vi "leapdata to fingers.vi"(11 "leapdata in":string="TYPE_THUMB0\nTYPE_INDEX72\nTYPE_MIDDLE67\nTYPE_RING57\nTYPE_PINKY59\n" caption="字符串/二进制数据") -> (1 "Recognize  hands":T1, 3 "fingerdata":T2)   [LabVIEW 2016]
uses:
  Controls/recognize hands data.ctl
panel:
  out "数字":i32[](array[numeric])
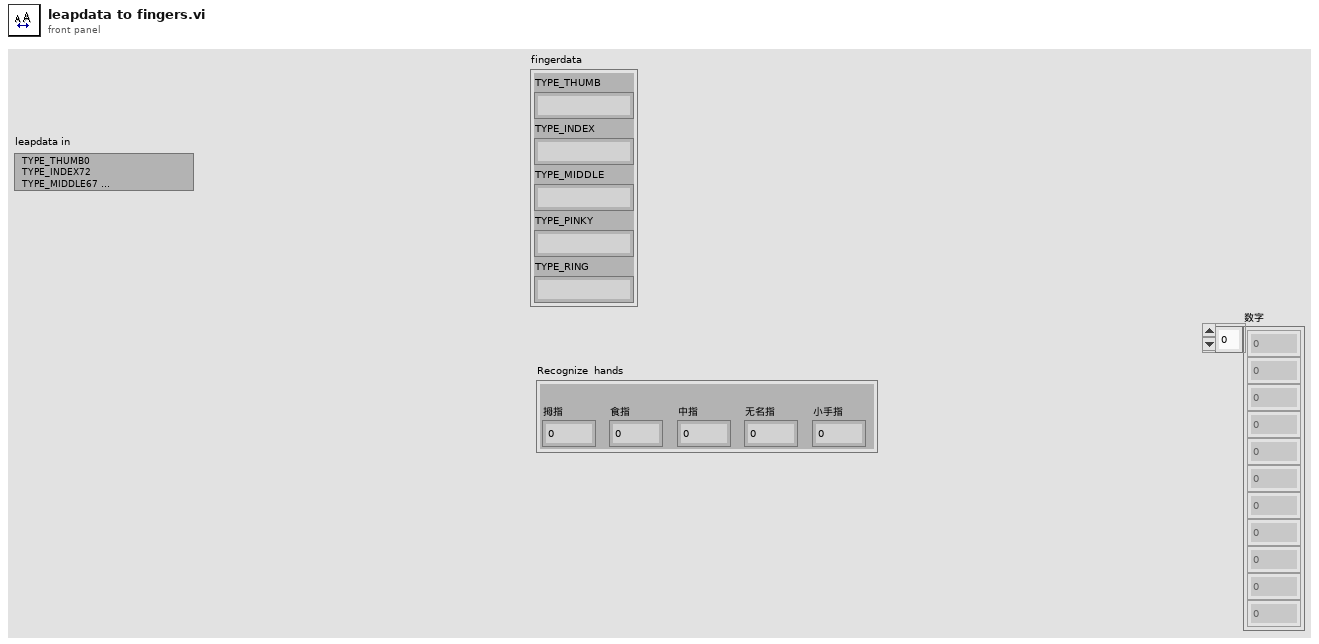
[diagram p1: front panel]
types:
  T1 = typedef "recognize hands data.ctl" = cluster{"小手指":sgl, "无名指":sgl, "中指":sgl, "食指":sgl, "拇指":sgl}
  T2 = cluster{"TYPE_THUMB":string, "TYPE_INDEX":string, "TYPE_MIDDLE":string, "TYPE_PINKY":string, "TYPE_RING":string}
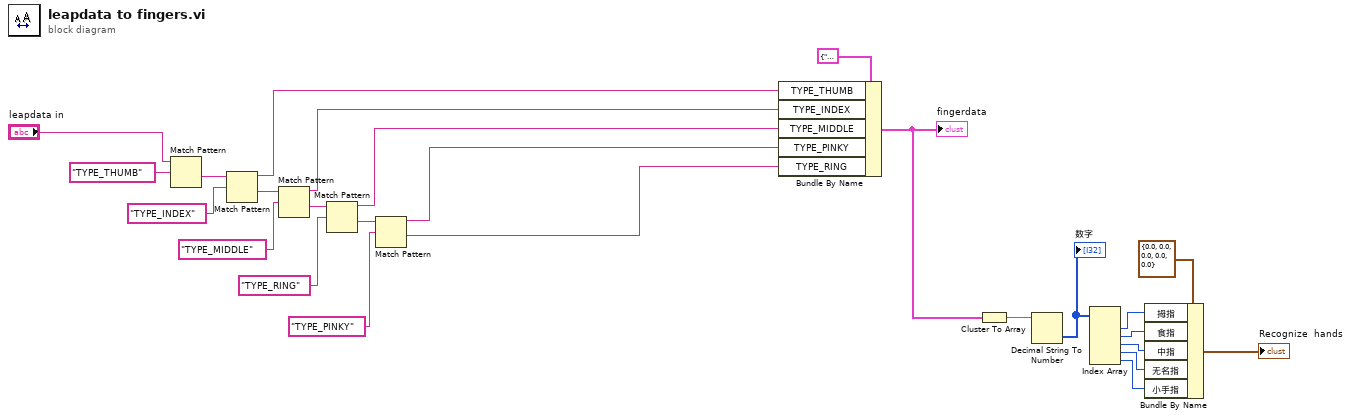
[diagram p0: block diagram]
diagram:
  n1 = Match Pattern(string="leapdata in", regular expression="TYPE_THUMB" ("搜索字符串")) -> (after substring=w24:string)  [unwired: 1 in, 3 out]
  n2 = Match Pattern(string=w24, regular expression="TYPE_INDEX" ("搜索字符串")) -> (before substring=w15:string, after substring=w22:string)  [unwired: 1 in, 2 out]
  n3 = Match Pattern(string=w22, regular expression="TYPE_MIDDLE" ("搜索字符串")) -> (before substring=w14:string, after substring=w20:string)  [unwired: 1 in, 2 out]
  n4 = Match Pattern(string=w20, regular expression="TYPE_RING" ("搜索字符串")) -> (before substring=w13:string, after substring=w18:string)  [unwired: 1 in, 2 out]
  n5 = Match Pattern(string=w18, regular expression="TYPE_PINKY" ("搜索字符串")) -> (before substring=w12:string, after substring=w11:string)  [unwired: 1 in, 2 out]
  n6 = Bundle By Name(cluster=T2 {"TYPE_THUMB"="0", "TYPE_INDEX"="81", "TYPE_MIDDLE"="82", "TYPE_PINKY"="72", "TYPE_RING"="75"}, "TYPE_THUMB"=w15, "TYPE_INDEX"=w14, "TYPE_MIDDLE"=w13, "TYPE_PINKY"=w12, "TYPE_RING"=w11) -> (w1:T2)
  "fingerdata" <- w1
  n7 = Cluster To Array(cluster=w1) -> (array=w10:string[])
  n8 = Decimal String To Number(string=w10) -> (number=w8:i32[])  [unwired: 2 in, 1 out]
  "数字" <- w8
  n9 = Index Array(array=w8) -> (element #1=w7:i32, element #2=w6:i32, element #3=w5:i32, element #4=w4:i32, element #5=w3:i32)  [unwired: 5 in]
  n10 = Bundle By Name(cluster=T1 {"小手指"=0.0, "无名指"=0.0, "中指"=0.0, "食指"=0.0, "拇指"=0.0} ("Reconze  hands"), "拇指"=w7, "食指"=w6, "中指"=w5, "无名指"=w4, "小手指"=w3) -> (→"Recognize  hands":T1)
